vi "Example NamedBundler 2.vi"() -> ()   [LabVIEW 2014]
panel:
  out "Double insideCluster":dbl
  out "LuboString":string
  out "Error Out":errorcluster
  in  "Error In":errorcluster
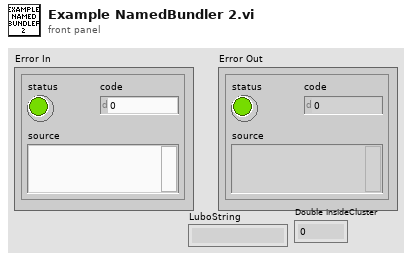
[diagram p1: front panel]
types:
  T1 = cluster{"DifferentTitle":string, "DifferentNumber":i32, "Different Double":dbl}
  T2 = cluster{"LuboString":string, "NumInsideUserCluter":i32, "Double insideCluster":dbl}
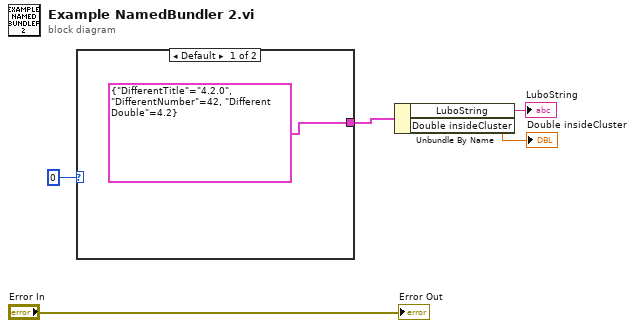
[diagram p0: block diagram]
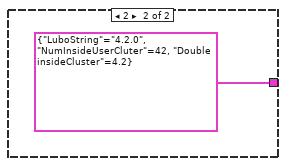
[diagram p2: hidden frame]
diagram:
  n1 = case shown="Default" 0 {
    tunnel: [T1 {"DifferentTitle"="4.2.0", "DifferentNumber"=42, "Different Double"=4.2} T2 {"LuboString"="4.2.0", "NumInsideUserCluter"=42, "Double insideCluster"=4.2}] -> w3
    frame Default {
    }
    frame 2 {
    }
  }
  n2 = Unbundle By Name(w3) -> ("LuboString"=→"LuboString":string, "Double insideCluster"=→"Double insideCluster":dbl)
  "Error Out" <- "Error In"
